vi "Execution timer.vi"(9 "error in (no error)":errorcluster, 10 "millisecond timer value":u32) -> (1 "error out":errorcluster, 2 "Current or Duration [ms]":u32)   [LabVIEW 2020, in "Support Utilities.lvlib"]
doc: "Returns the current time in milliseconds if the input is not wired.\nIf the input is wired the time differens is returned in milliseconds."
uses:
  Support Utilities.lvlib
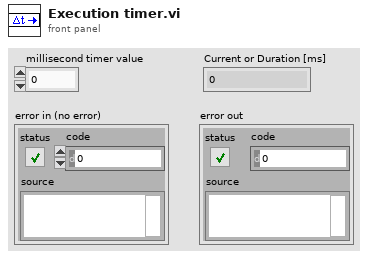
[diagram p1: front panel]
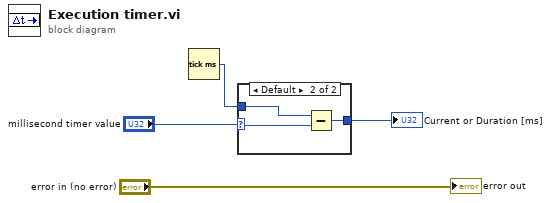
[diagram p0: block diagram]
diagram:
  n1 = Tick Count (ms)() -> (millisecond timer value=w1:u32)
  n2 = case shown="Default" "millisecond timer value" {
    selector: "millisecond timer value" -> [_ w8]
    tunnel: w1 -> [w5 w7]
    tunnel: [w5 w6] -> w2
    frame 0 {
    }
    frame Default {
      n3 = Subtract(x=w7, y=w8) -> (x-y=w6:u32)
    }
  }
  "Current or Duration [ms]" <- w2
  "error out" <- "error in (no error)"
